vi "IdontKnow.vi"   [LabVIEW 2017]
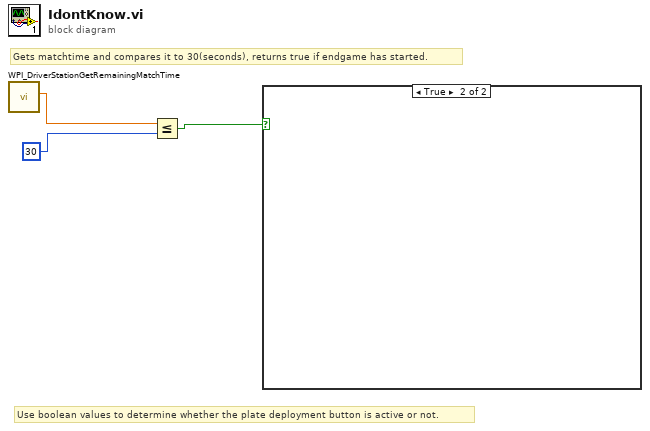
[diagram p0: block diagram]
diagram:
  # "Use boolean values to determine whether the plate deployment button is active or not."
  # "Gets matchtime and compares it to 30(seconds), returns true if endgame has started."
  n1 = call <vilib>:"WPI_DriverStationGetRemainingMatchTime.vi"() -> ("Match Time(s)"=w2:sgl)  [unwired: 10 in, 1 out]
  n2 = Less Or Equal?(x=w2, y=30) -> (x <= y?=w1:bool)
  n3 = case shown="True" w1 {
    frame False {
    }
    frame True {
    }
  }
